vi "AlGaInPAs_v19d.vi"(2 "Debug Mode":bool, 3 "Elapsed Time(s)":dbl, 4 "State":enum16{"Edit", "Start", "Run", "End", "Idle"}(ring), 5 "Argument List In":string[](array[string])) -> (0 "Status Out":string, 1 "Argument List Out":string[](array[string]))   [LabVIEW 2011]
panel:
  out "P bubbler Copy":T1 {"P bubbler main"."Flow" format="%.2f"}
  out "P bubbler":T1 {"P bubbler main"."Flow" format="%.2f"}
  out "As gas Copy":T2 {"As gas main"."Flow" format="%.2f"}
  out "As gas":T2 {"As gas main"."Flow" format="%.2f"}
  out "P gas Copy":T3 {"P gas main"."Flow" format="%.2f"}
  out "P gas":T3 {"P gas main"."Flow" format="%.2f"}
  out "In bubbler Copy":T4 {"In main"."Flow" format="%.2f"}
  in  "In bubbler":T4 {"In main"."Flow" format="%.2f"}
  out "Ga bubbler Copy":T5={"Ga bubbler Active"=FALSE, "Ga main"={"Flow"=0.0, "Ga Run"=FALSE, "Prep Ga"=FALSE, "Dilution"=FALSE, "Ga Calculated"=1, "MFC2 flow"=10.0, "MFC3 flow"=100.0, "MFC1 flow"=0.0}} {"Ga main"."MFC1 flow" format="%.4f"; "Ga main"."MFC3 flow" format="%.1f"; "Ga main"."MFC2 flow" format="%.2f"; "Ga main"."Ga Calculated" items=["Ga flow", "MFC1", "MFC2", "MFC3"]; "Ga main"."Flow" format="%.2f"}
  out "Ga bubbler":T5={"Ga bubbler Active"=FALSE, "Ga main"={"Flow"=0.0, "Ga Run"=FALSE, "Prep Ga"=FALSE, "Dilution"=FALSE, "Ga Calculated"=1, "MFC2 flow"=10.0, "MFC3 flow"=100.0, "MFC1 flow"=0.0}} {"Ga main"."MFC1 flow" format="%.4f"; "Ga main"."MFC3 flow" format="%.1f"; "Ga main"."MFC2 flow" format="%.2f"; "Ga main"."Ga Calculated" items=["Ga flow", "MFC1", "MFC2", "MFC3"]; "Ga main"."Flow" format="%.2f"}
  out "Al bubbler Copy":T6 {"Al main"."Al Flow" format="%.2f"}
  out "Al bubbler":T6 {"Al main"."Al Flow" format="%.2f"}
  out "prep_done":bool
  out "run started":bool
  out "first":bool=TRUE
  out "total time":dbl
  out "is OK?":bool
  in  "prep_time":dbl
  in  "Cancel":bool
  in  "OK":bool
  out "tTotal(s) 2":dbl
  # "Add pre-run time to run time in editor."
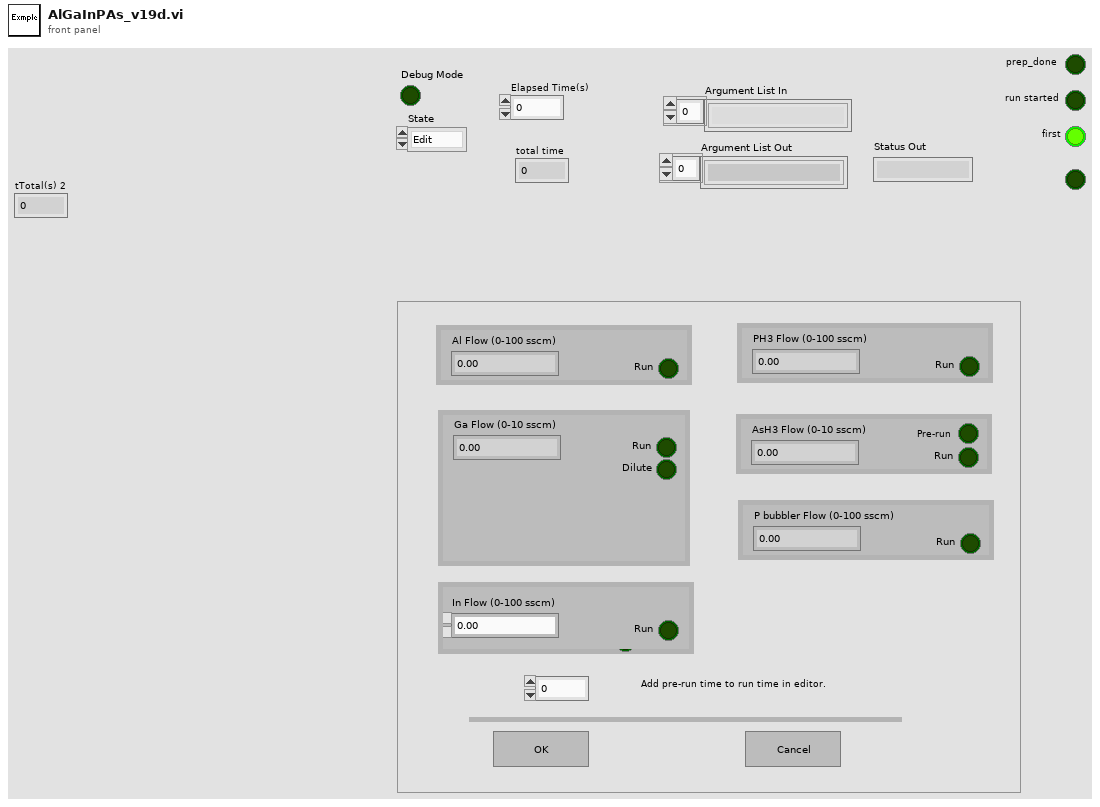
[diagram p1: front panel]
types:
  T1 = cluster{"P bubbler Active":bool, "P bubbler main":cluster{"Flow":dbl, "P bubbler Run":bool, "P bubbler Prep":bool}}
  T2 = cluster{"As gas Active":bool, "As gas main":cluster{"Flow":dbl, "AsH3 Run":bool, "AsH3 Prep":bool}}
  T3 = cluster{"P gas Active":bool, "P gas main":cluster{"Flow":dbl, "PH3 Run":bool, "PH3 Prep":bool}}
  T4 = cluster{"In main":cluster{"Flow":dbl, "In Run":bool, "Prep In":bool}, "In bubbler Active":bool}
  T5 = cluster{"Ga bubbler Active":bool, "Ga main":cluster{"Flow":dbl, "Ga Run":bool, "Prep Ga":bool, "Dilution":bool, "Ga Calculated":u16, "MFC2 flow":dbl, "MFC3 flow":dbl, "MFC1 flow":dbl}}
  T6 = cluster{"Al Active":bool, "Al main":cluster{"Al Flow":dbl, "Al Run":bool, "Prep Al":bool}}
  T7 = enum16{"Discrete", "Continuous", "Instantaneous", "Finite"}
  T8 = enum32{"Invalid", "Default", "Floating", "Floating/Auto-Hide", "Modal"}
  T9 = enum8{"Enabled", "Disabled", "Disabled and Grayed Out"}
  T10 = cluster{"Al Flow":dbl, "Al Run":bool, "Prep Al":bool}
  T11 = cluster{"Flow":dbl, "Ga Run":bool, "Prep Ga":bool, "Dilution":bool, "Ga Calculated":u16, "MFC2 flow":dbl, "MFC3 flow":dbl, "MFC1 flow":dbl}
  T12 = cluster{"Flow":dbl, "In Run":bool, "Prep In":bool}
  T13 = cluster{"Flow":dbl, "PH3 Run":bool, "PH3 Prep":bool}
  T14 = cluster{"Flow":dbl, "AsH3 Run":bool, "AsH3 Prep":bool}
  T15 = cluster{"Flow":dbl, "P bubbler Run":bool, "P bubbler Prep":bool}
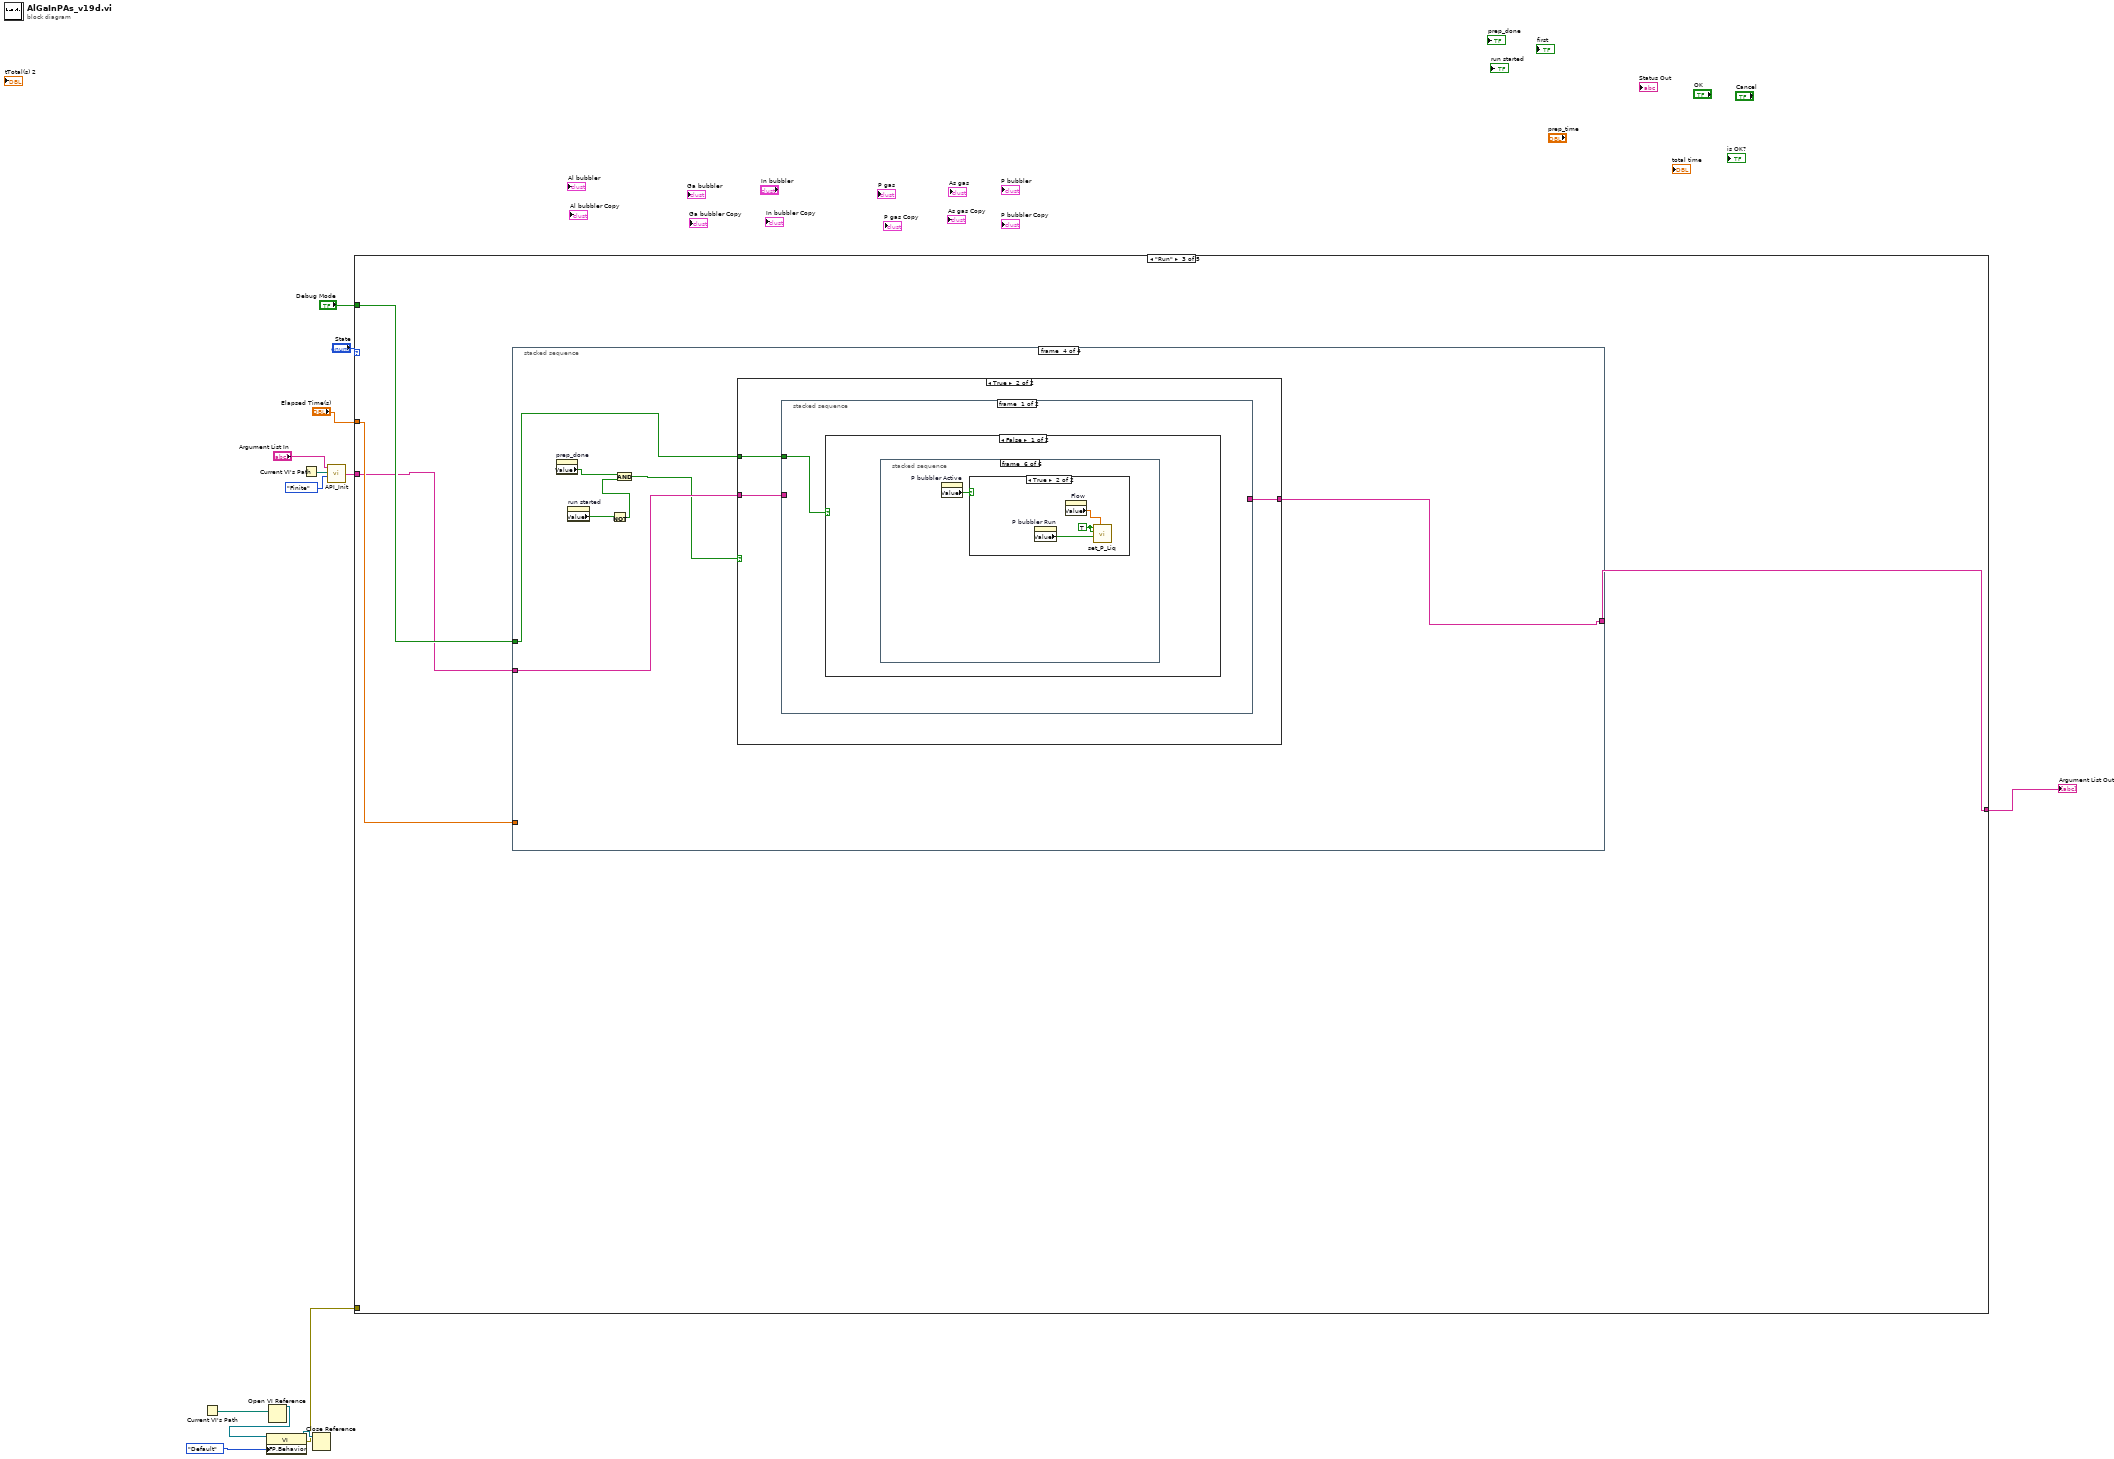
[diagram p0: block diagram]
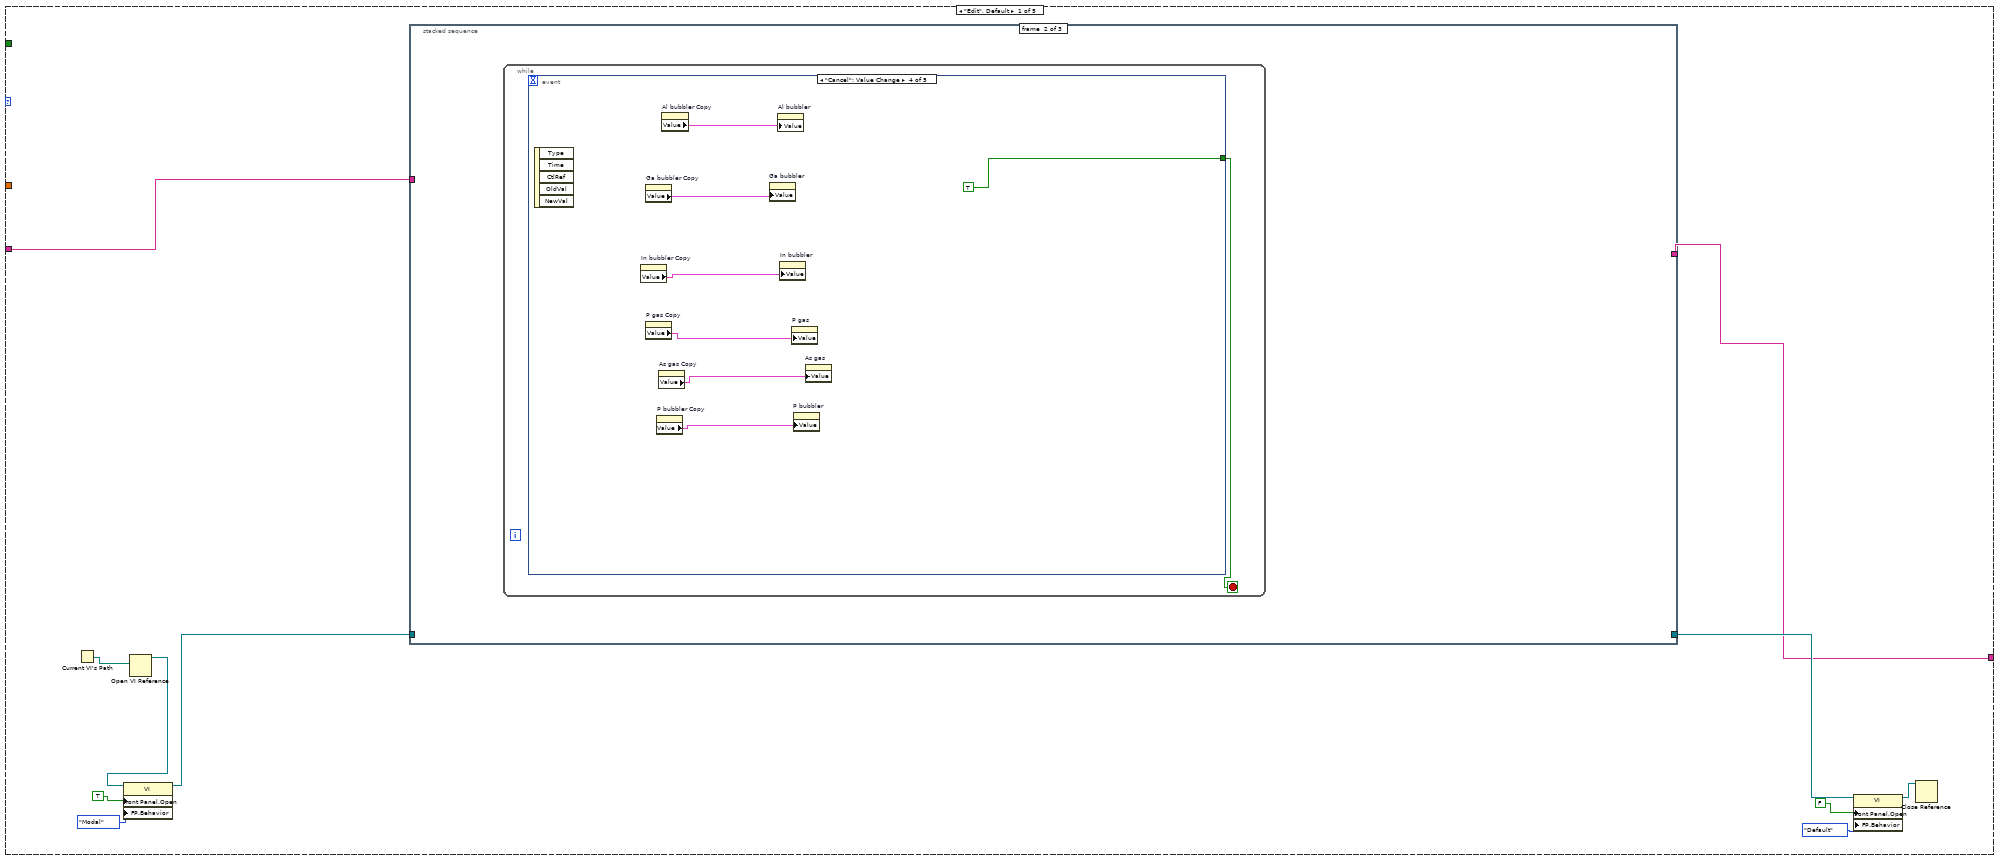
[diagram p2: hidden frame]
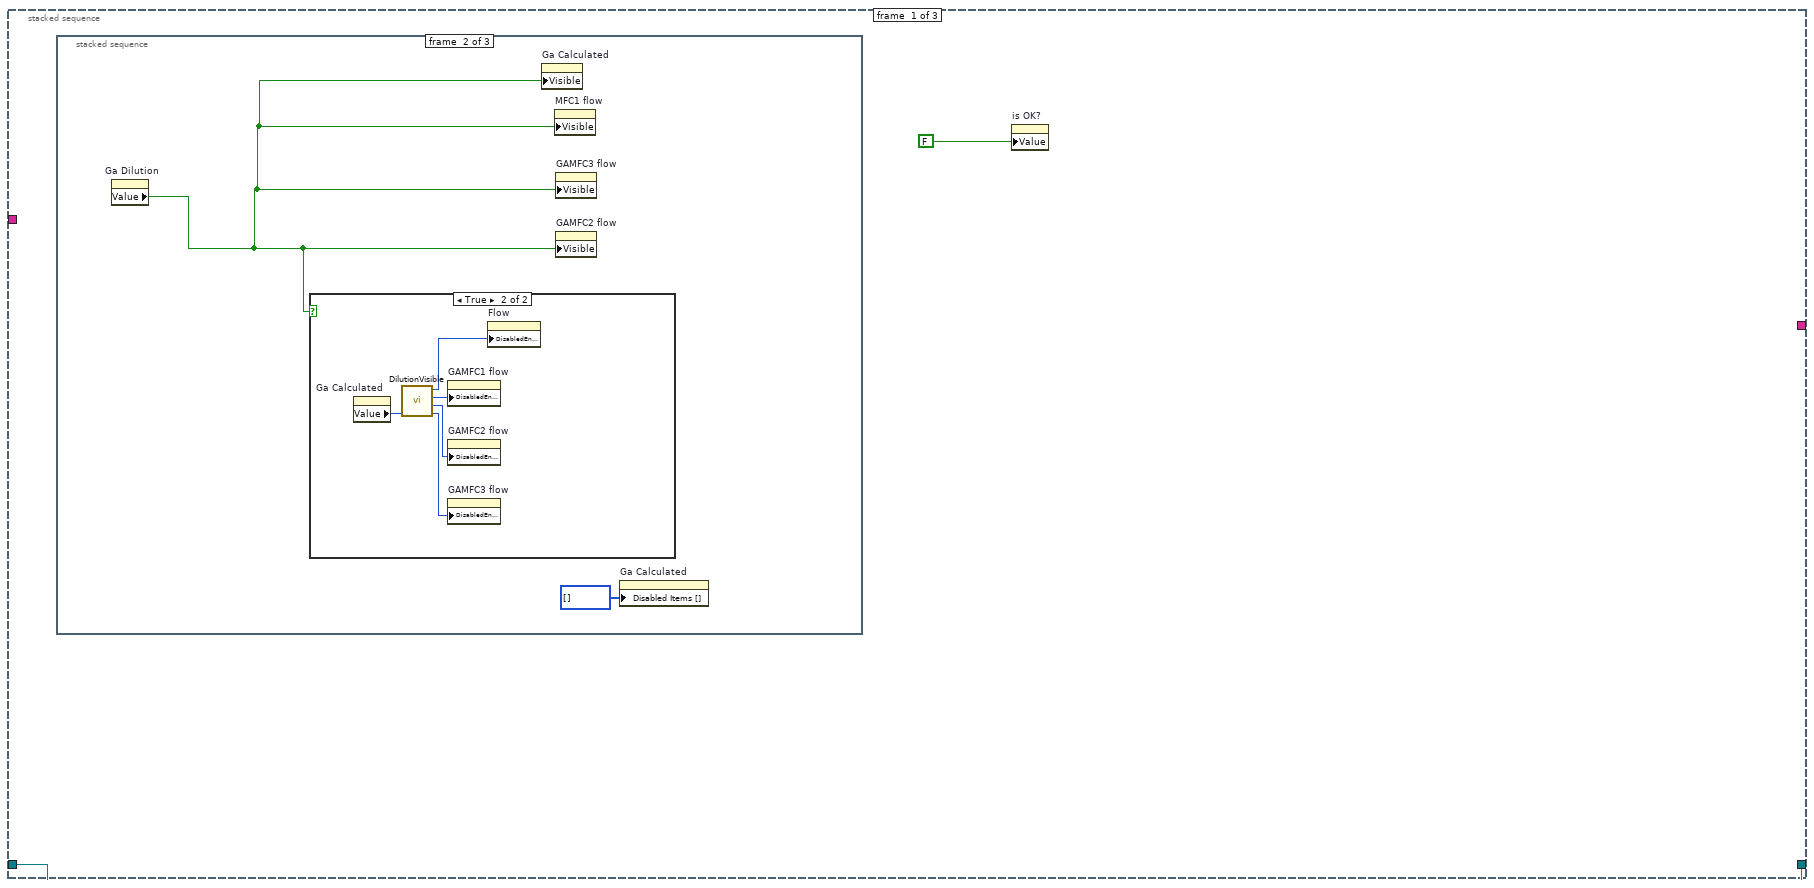
[diagram p3: hidden frame]
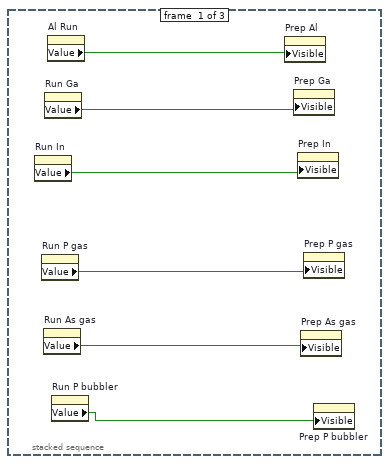
[diagram p4: hidden frame]
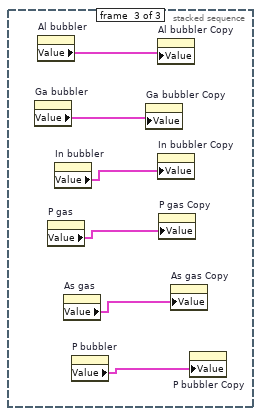
[diagram p6: hidden frame]
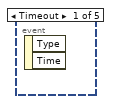
[diagram p7: hidden frame]
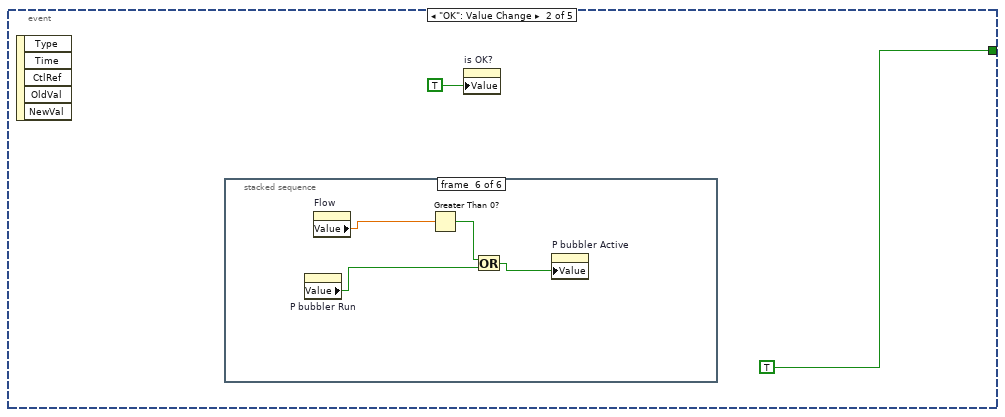
[diagram p8: hidden frame]
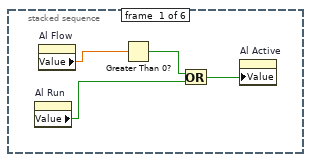
[diagram p9: hidden frame]
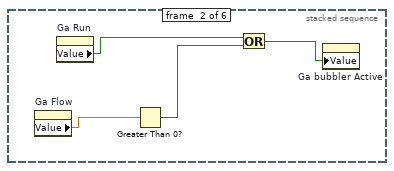
[diagram p10: hidden frame]
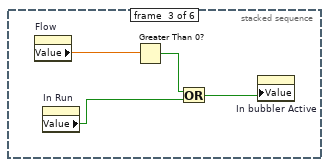
[diagram p11: hidden frame]
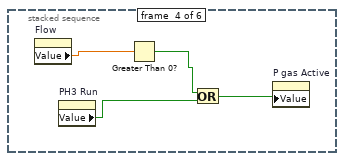
[diagram p12: hidden frame]
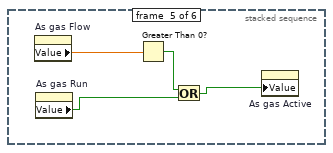
[diagram p13: hidden frame]
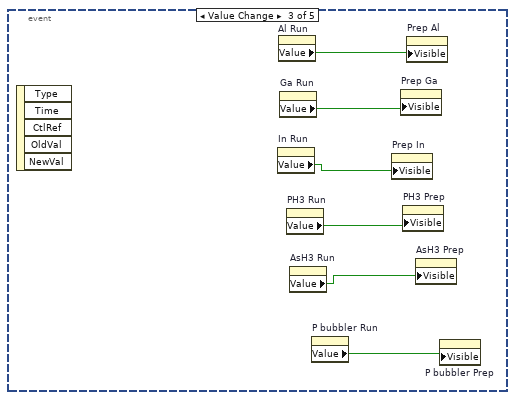
[diagram p14: hidden frame]
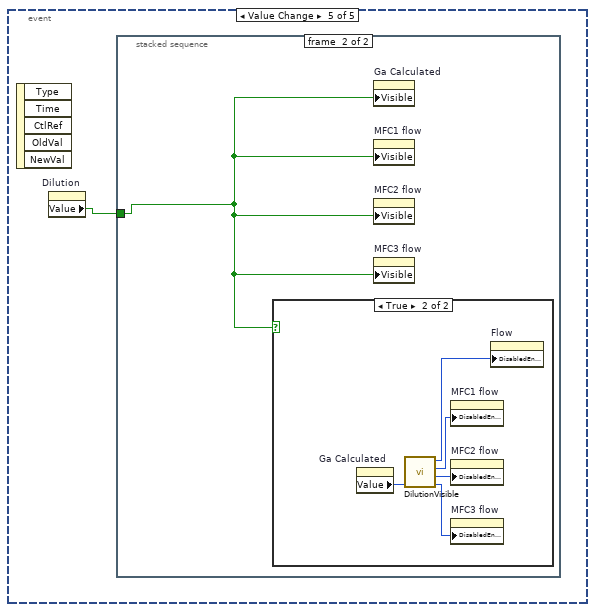
[diagram p15: hidden frame]
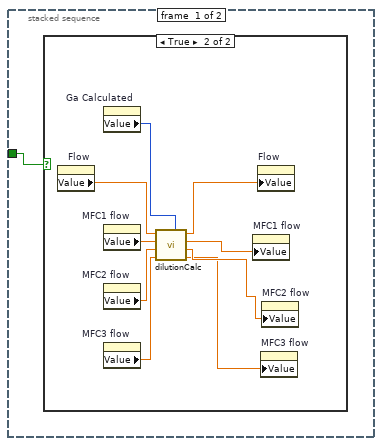
[diagram p16: hidden frame]
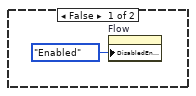
[diagram p18: hidden frame]
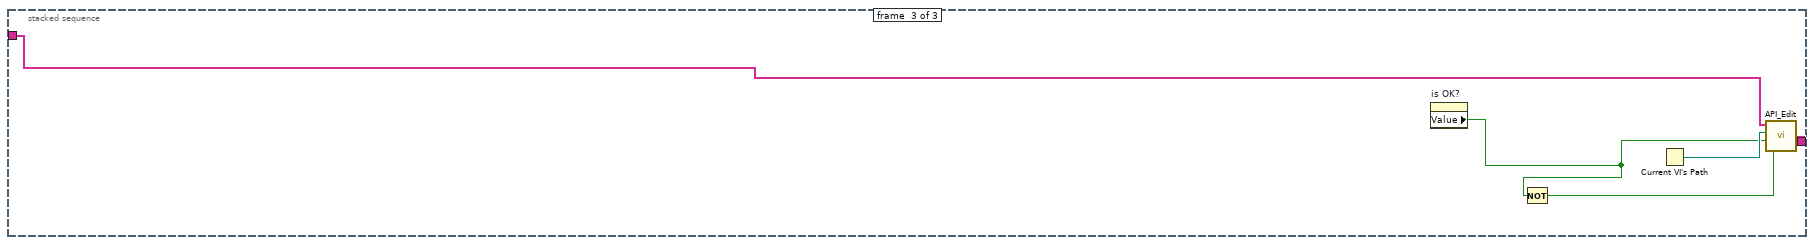
[diagram p19: hidden frame]
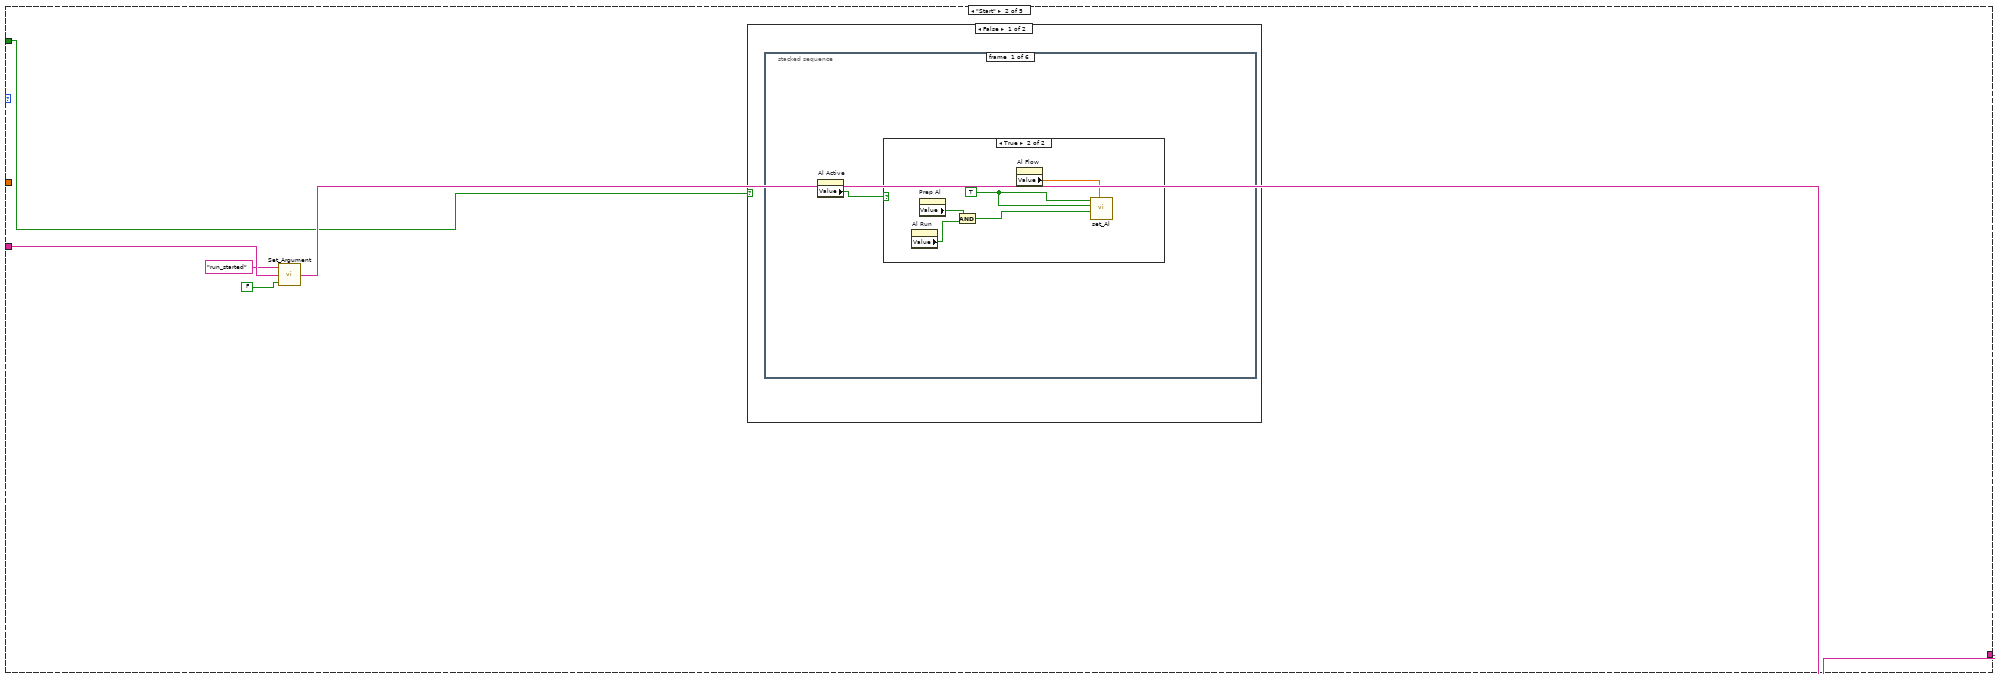
[diagram p20: hidden frame]
diagram:
  n1 = Current VI's Path() -> (path=w9:path)
  n2 = Open VI Reference(vi path=w9) -> (vi reference=w8:refnum<vi>)  [unwired: 1 in, 5 out]
  n3 = property class="VI"(reference=w8, "FP.Behavior"=T8."Default" ("Front Panel Window:Behavior")) -> (reference out=w6:refnum<vi>, error out=w5:errorcluster)  [unwired: 1 in]
  n4 = Current VI's Path() -> (path=w4:path)
  n5 = Close Reference(reference=w6) -> ()  [unwired: 1 in, 1 out]
  n6 = call "API_Init.vi"("API Mode"=T7."Finite", "VI Path"=w4, "Argument List In"="Argument List In") -> ("Argument List Out"=w1:string[])  [unwired: 1 in]
  n7 = case shown="\"Run\"" "State" {
    tunnel: "Debug Mode" -> [_ w109 w167 _ _]
    tunnel: "Elapsed Time(s)" -> [_ _ w168 _ _]
    tunnel: w1 -> [w15 w111 w166 w297 w298]
    tunnel: [w14 w110 w165 w297 w298] -> w10
    tunnel: w5 -> [_ _ _ _ _]
    frame "Edit", Default {
      n8 = Current VI's Path() -> (path=w20:path)
      n9 = Open VI Reference(vi path=w20) -> (vi reference=w19:refnum<vi>)  [unwired: 1 in, 5 out]
      n10 = property class="VI"(reference=w19, "Front Panel.Open"=TRUE ("Front Panel Window:Open"), "FP.Behavior"=T8."Modal" ("Front Panel Window:Behavior")) -> (reference out=w18:refnum<vi>)  [unwired: 1 in, 1 out]
      n11 = stacked-sequence {
        tunnel: w15 -> [_ _ w105]
        tunnel: w18 -> [w26 _ _]
        tunnel: [w26 _ _] -> w22
        tunnel: [_ _ w106] -> w14
        frame #0 {
          n12 = stacked-sequence {
            frame #0 {
              n13 = property on="Run In" class="Bool (strict)"() -> ("Value"=w31:bool)  [unwired: 2 in, 2 out]
              n14 = property on="Run P gas" class="Bool (strict)"() -> ("Value"=w29:bool)  [unwired: 2 in, 2 out]
              n15 = property on="Run As gas" class="Bool (strict)"() -> ("Value"=w28:bool)  [unwired: 2 in, 2 out]
              n16 = property on="Run Ga" class="Bool (strict)"() -> ("Value"=w30:bool)  [unwired: 2 in, 2 out]
              n17 = property on="Al Run" class="Bool (strict)"() -> ("Value"=w32:bool)  [unwired: 2 in, 2 out]
              n18 = property on="Run P bubbler" class="Bool (strict)"() -> ("Value"=w27:bool)  [unwired: 2 in, 2 out]
              n19 = property on="Prep Al" class="Bool (strict)"("Visible"=w32) -> ()  [unwired: 2 in, 2 out]
              n20 = property on="Prep Ga" class="Bool (strict)"("Visible"=w30) -> ()  [unwired: 2 in, 2 out]
              n21 = property on="Prep In" class="Bool (strict)"("Visible"=w31) -> ()  [unwired: 2 in, 2 out]
              n22 = property on="Prep As gas" class="Bool (strict)"("Visible"=w28) -> ()  [unwired: 2 in, 2 out]
              n23 = property on="Prep P gas" class="Bool (strict)"("Visible"=w29) -> ()  [unwired: 2 in, 2 out]
              n24 = property on="Prep P bubbler" class="Bool (strict)"("Visible"=w27) -> ()  [unwired: 2 in, 2 out]
            }
            frame #1 {
              n25 = property on="Ga Dilution" class="Bool (strict)"() -> ("Value"=w34:bool)  [unwired: 2 in, 2 out]
              n26 = case shown="True" w34 {
                frame False {
                }
                frame True {
                  n27 = property on="Ga Calculated" class="Ring (strict)"() -> ("Value"=w35:u16)  [unwired: 2 in, 2 out]
                  n28 = call "DilutionVisible.vi"("calculated"=w35) -> ("MFC3"=w38:u16, "MFC2"=w37:u16, "MFC1"=w36:u16, "flow"=w39:u16)  [unwired: 3 in]
                  n29 = property on="GAMFC1 flow" class="DigNum (strict)"("DisabledEnum"=w36) -> ()  [unwired: 2 in, 2 out]
                  n30 = property on="GAMFC2 flow" class="DigNum (strict)"("DisabledEnum"=w37) -> ()  [unwired: 2 in, 2 out]
                  n31 = property on="GAMFC3 flow" class="DigNum (strict)"("DisabledEnum"=w38) -> ()  [unwired: 2 in, 2 out]
                  n32 = property on="Flow" class="DigNum (strict)"("DisabledEnum"=w39) -> ()  [unwired: 2 in, 2 out]
                }
              }
              n33 = property on="Ga Calculated" class="Ring (strict)"("Visible"=w34) -> ()  [unwired: 2 in, 2 out]
              n34 = property on="MFC1 flow" class="DigNum (strict)"("Visible"=w34) -> ()  [unwired: 2 in, 2 out]
              n35 = property on="GAMFC3 flow" class="DigNum (strict)"("Visible"=w34) -> ()  [unwired: 2 in, 2 out]
              n36 = property on="GAMFC2 flow" class="DigNum (strict)"("Visible"=w34) -> ()  [unwired: 2 in, 2 out]
              n37 = property on="Ga Calculated" class="Ring (strict)"("Disabled Items []"=i32[] []) -> ()  [unwired: 2 in, 2 out]
            }
            frame #2 {
              n38 = property on="Ga bubbler" class="Clust (strict)"() -> ("Value"=w44:T5)  [unwired: 2 in, 2 out]
              n39 = property on="Al bubbler" class="Clust (strict)"() -> ("Value"=w45:T6)  [unwired: 2 in, 2 out]
              n40 = property on="P gas" class="Clust (strict)"() -> ("Value"=w42:T3)  [unwired: 2 in, 2 out]
              n41 = property on="In bubbler" class="Clust (strict)"() -> ("Value"=w43:T4)  [unwired: 2 in, 2 out]
              n42 = property on="As gas" class="Clust (strict)"() -> ("Value"=w41:T2)  [unwired: 2 in, 2 out]
              n43 = property on="P bubbler" class="Clust (strict)"() -> ("Value"=w40:T1)  [unwired: 2 in, 2 out]
              n44 = property on="Ga bubbler Copy" class="Clust (strict)"("Value"=w44) -> ()  [unwired: 2 in, 2 out]
              n45 = property on="Al bubbler Copy" class="Clust (strict)"("Value"=w45) -> ()  [unwired: 2 in, 2 out]
              n46 = property on="In bubbler Copy" class="Clust (strict)"("Value"=w43) -> ()  [unwired: 2 in, 2 out]
              n47 = property on="P gas Copy" class="Clust (strict)"("Value"=w42) -> ()  [unwired: 2 in, 2 out]
              n48 = property on="As gas Copy" class="Clust (strict)"("Value"=w41) -> ()  [unwired: 2 in, 2 out]
              n49 = property on="P bubbler Copy" class="Clust (strict)"("Value"=w40) -> ()  [unwired: 2 in, 2 out]
            }
          }
          n50 = property on="is OK?" class="Bool (strict)"("Value"=FALSE ("is OK?")) -> ()  [unwired: 2 in, 2 out]
        }
        frame #1 {
          n51 = while {
            stop <- w46 stop-if-true
            n52 = event shown="[3] \"Cancel\": Value Change" {
              selector: _ -> [_ _ _ _ _]
              dyn-events: _ -> [_ _ _ _ _]
              timeout: _ -> [_ _ _ _ _]
              tunnel: [_ TRUE _ TRUE _] -> w46
              event Timeout {
                n53 = event-data() -> ()  [unwired: 1 in, 2 out]
              }
              event "OK": Value Change {
                n54 = event-data() -> ()  [unwired: 1 in, 5 out]
                n55 = stacked-sequence {
                  frame #0 {
                    n56 = property on="Al Run" class="Bool (strict)"() -> ("Value"=w50:bool)  [unwired: 2 in, 2 out]
                    n57 = property on="Al Flow" class="DigNum (strict)"() -> ("Value"=w51:dbl)  [unwired: 2 in, 2 out]
                    n58 = Greater Than 0?(x=w51) -> (x > 0?=w52:bool)
                    n59 = Or(x=w52, y=w50) -> (x .or. y?=w49:bool)
                    n60 = property on="Al Active" class="Bool (strict)"("Value"=w49) -> ()  [unwired: 2 in, 2 out]
                  }
                  frame #1 {
                    n61 = property on="Ga Flow" class="DigNum (strict)"() -> ("Value"=w53:dbl)  [unwired: 2 in, 2 out]
                    n62 = property on="Ga Run" class="Bool (strict)"() -> ("Value"=w54:bool)  [unwired: 2 in, 2 out]
                    n63 = Greater Than 0?(x=w53) -> (x > 0?=w56:bool)
                    n64 = Or(x=w54, y=w56) -> (x .or. y?=w55:bool)
                    n65 = property on="Ga bubbler Active" class="Bool (strict)"("Value"=w55) -> ()  [unwired: 2 in, 2 out]
                  }
                  frame #2 {
                    n66 = property on="Flow" class="DigNum (strict)"() -> ("Value"=w59:dbl)  [unwired: 2 in, 2 out]
                    n67 = property on="In Run" class="Bool (strict)"() -> ("Value"=w58:bool)  [unwired: 2 in, 2 out]
                    n68 = Greater Than 0?(x=w59) -> (x > 0?=w60:bool)
                    n69 = Or(x=w60, y=w58) -> (x .or. y?=w57:bool)
                    n70 = property on="In bubbler Active" class="Bool (strict)"("Value"=w57) -> ()  [unwired: 2 in, 2 out]
                  }
                  frame #3 {
                    n71 = property on="Flow" class="DigNum (strict)"() -> ("Value"=w63:dbl)  [unwired: 2 in, 2 out]
                    n72 = property on="PH3 Run" class="Bool (strict)"() -> ("Value"=w62:bool)  [unwired: 2 in, 2 out]
                    n73 = Greater Than 0?(x=w63) -> (x > 0?=w64:bool)
                    n74 = Or(x=w64, y=w62) -> (x .or. y?=w61:bool)
                    n75 = property on="P gas Active" class="Bool (strict)"("Value"=w61) -> ()  [unwired: 2 in, 2 out]
                  }
                  frame #4 {
                    n76 = property on="As gas Flow" class="DigNum (strict)"() -> ("Value"=w67:dbl)  [unwired: 2 in, 2 out]
                    n77 = property on="As gas Run" class="Bool (strict)"() -> ("Value"=w66:bool)  [unwired: 2 in, 2 out]
                    n78 = Greater Than 0?(x=w67) -> (x > 0?=w68:bool)
                    n79 = Or(x=w68, y=w66) -> (x .or. y?=w65:bool)
                    n80 = property on="As gas Active" class="Bool (strict)"("Value"=w65) -> ()  [unwired: 2 in, 2 out]
                  }
                  frame #5 {
                    n81 = property on="P bubbler Run" class="Bool (strict)"() -> ("Value"=w70:bool)  [unwired: 2 in, 2 out]
                    n82 = property on="Flow" class="DigNum (strict)"() -> ("Value"=w71:dbl)  [unwired: 2 in, 2 out]
                    n83 = Greater Than 0?(x=w71) -> (x > 0?=w72:bool)
                    n84 = Or(x=w72, y=w70) -> (x .or. y?=w69:bool)
                    n85 = property on="P bubbler Active" class="Bool (strict)"("Value"=w69) -> ()  [unwired: 2 in, 2 out]
                  }
                }
                n86 = property on="is OK?" class="Bool (strict)"("Value"=TRUE ("is OK?")) -> ()  [unwired: 2 in, 2 out]
              }
              event "Ga bubbler.Ga main.Ga Run", "In bubbler.In main.In Run", "P gas.P gas main.PH3 Run", "As gas.As gas main.AsH3 Run", "Al bubbler.Al main.Al Run", "P bubbler.P bubbler main.P bubbler Run": Value Change {
                n87 = event-data() -> ()  [unwired: 1 in, 5 out]
                n88 = property on="In Run" class="Bool (strict)"() -> ("Value"=w75:bool)  [unwired: 2 in, 2 out]
                n89 = property on="Al Run" class="Bool (strict)"() -> ("Value"=w77:bool)  [unwired: 2 in, 2 out]
                n90 = property on="Ga Run" class="Bool (strict)"() -> ("Value"=w76:bool)  [unwired: 2 in, 2 out]
                n91 = property on="PH3 Run" class="Bool (strict)"() -> ("Value"=w74:bool)  [unwired: 2 in, 2 out]
                n92 = property on="AsH3 Run" class="Bool (strict)"() -> ("Value"=w73:bool)  [unwired: 2 in, 2 out]
                n93 = property on="P bubbler Run" class="Bool (strict)"() -> ("Value"=w78:bool)  [unwired: 2 in, 2 out]
                n94 = property on="Prep In" class="Bool (strict)"("Visible"=w75) -> ()  [unwired: 2 in, 2 out]
                n95 = property on="Prep Ga" class="Bool (strict)"("Visible"=w76) -> ()  [unwired: 2 in, 2 out]
                n96 = property on="PH3 Prep" class="Bool (strict)"("Visible"=w74) -> ()  [unwired: 2 in, 2 out]
                n97 = property on="Prep Al" class="Bool (strict)"("Visible"=w77) -> ()  [unwired: 2 in, 2 out]
                n98 = property on="AsH3 Prep" class="Bool (strict)"("Visible"=w73) -> ()  [unwired: 2 in, 2 out]
                n99 = property on="P bubbler Prep" class="Bool (strict)"("Visible"=w78) -> ()  [unwired: 2 in, 2 out]
              }
              event "Cancel": Value Change {
                n100 = event-data() -> ()  [unwired: 1 in, 5 out]
                n101 = property on="In bubbler Copy" class="Clust (strict)"() -> ("Value"=w83:T4)  [unwired: 2 in, 2 out]
                n102 = property on="Ga bubbler Copy" class="Clust (strict)"() -> ("Value"=w82:T5)  [unwired: 2 in, 2 out]
                n103 = property on="P gas Copy" class="Clust (strict)"() -> ("Value"=w81:T3)  [unwired: 2 in, 2 out]
                n104 = property on="P bubbler Copy" class="Clust (strict)"() -> ("Value"=w79:T1)  [unwired: 2 in, 2 out]
                n105 = property on="As gas Copy" class="Clust (strict)"() -> ("Value"=w80:T2)  [unwired: 2 in, 2 out]
                n106 = property on="Al bubbler Copy" class="Clust (strict)"() -> ("Value"=w84:T6)  [unwired: 2 in, 2 out]
                n107 = property on="Ga bubbler" class="Clust (strict)"("Value"=w82) -> ()  [unwired: 2 in, 2 out]
                n108 = property on="Al bubbler" class="Clust (strict)"("Value"=w84) -> ()  [unwired: 2 in, 2 out]
                n109 = property on="In bubbler" class="Clust (strict)"("Value"=w83) -> ()  [unwired: 2 in, 2 out]
                n110 = property on="P gas" class="Clust (strict)"("Value"=w81) -> ()  [unwired: 2 in, 2 out]
                n111 = property on="P bubbler" class="Clust (strict)"("Value"=w79) -> ()  [unwired: 2 in, 2 out]
                n112 = property on="As gas" class="Clust (strict)"("Value"=w80) -> ()  [unwired: 2 in, 2 out]
              }
              event "Ga bubbler.Ga main.Ga Calculated", "Ga bubbler.Ga main.MFC1 flow", "Ga bubbler.Ga main.MFC2 flow", "Ga bubbler.Ga main.MFC3 flow", "Ga bubbler.Ga main.Flow", "Ga bubbler.Ga main.Dilution": Value Change {
                n113 = event-data() -> ()  [unwired: 1 in, 5 out]
                n114 = property on="Dilution" class="Bool (strict)"() -> ("Value"=w86:bool)  [unwired: 2 in, 2 out]
                n115 = stacked-sequence {
                  tunnel: w86 -> [w87 w97]
                  frame #0 {
                    n116 = case shown="True" w87 {
                      frame False {
                      }
                      frame True {
                        n117 = property on="Flow" class="DigNum (strict)"() -> ("Value"=w95:dbl)  [unwired: 2 in, 2 out]
                        n118 = property on="Ga Calculated" class="Ring (strict)"() -> ("Value"=w96:u16)  [unwired: 2 in, 2 out]
                        n119 = property on="MFC1 flow" class="DigNum (strict)"() -> ("Value"=w94:dbl)  [unwired: 2 in, 2 out]
                        n120 = property on="MFC2 flow" class="DigNum (strict)"() -> ("Value"=w93:dbl)  [unwired: 2 in, 2 out]
                        n121 = property on="MFC3 flow" class="DigNum (strict)"() -> ("Value"=w92:dbl)  [unwired: 2 in, 2 out]
                        n122 = call "dilutionCalc.vi"("Calculated"=w96, "MFC3"=w92, "MFC2"=w93, "MFC1"=w94, "flow"=w95) -> ("MFC3 out"=w88:dbl, "MFC2 out"=w89:dbl, "MFC1 out"=w90:dbl, "flow out"=w91:dbl)  [unwired: 1 in]
                        n123 = property on="MFC1 flow" class="DigNum (strict)"("Value"=w90) -> ()  [unwired: 2 in, 2 out]
                        n124 = property on="Flow" class="DigNum (strict)"("Value"=w91) -> ()  [unwired: 2 in, 2 out]
                        n125 = property on="MFC3 flow" class="DigNum (strict)"("Value"=w88) -> ()  [unwired: 2 in, 2 out]
                        n126 = property on="MFC2 flow" class="DigNum (strict)"("Value"=w89) -> ()  [unwired: 2 in, 2 out]
                      }
                    }
                  }
                  frame #1 {
                    n127 = case shown="True" w97 {
                      frame False {
                        n128 = property on="Flow" class="DigNum (strict)"("DisabledEnum"=T9."Enabled" ("Disabled")) -> ()  [unwired: 2 in, 2 out]
                      }
                      frame True {
                        n129 = property on="Ga Calculated" class="Ring (strict)"() -> ("Value"=w99:u16)  [unwired: 2 in, 2 out]
                        n130 = call "DilutionVisible.vi"("calculated"=w99) -> ("MFC3"=w103:u16, "MFC2"=w102:u16, "MFC1"=w101:u16, "flow"=w100:u16)  [unwired: 3 in]
                        n131 = property on="MFC1 flow" class="DigNum (strict)"("DisabledEnum"=w101) -> ()  [unwired: 2 in, 2 out]
                        n132 = property on="MFC2 flow" class="DigNum (strict)"("DisabledEnum"=w102) -> ()  [unwired: 2 in, 2 out]
                        n133 = property on="MFC3 flow" class="DigNum (strict)"("DisabledEnum"=w103) -> ()  [unwired: 2 in, 2 out]
                        n134 = property on="Flow" class="DigNum (strict)"("DisabledEnum"=w100) -> ()  [unwired: 2 in, 2 out]
                      }
                    }
                    n135 = property on="Ga Calculated" class="Ring (strict)"("Visible"=w97) -> ()  [unwired: 2 in, 2 out]
                    n136 = property on="MFC1 flow" class="DigNum (strict)"("Visible"=w97) -> ()  [unwired: 2 in, 2 out]
                    n137 = property on="MFC2 flow" class="DigNum (strict)"("Visible"=w97) -> ()  [unwired: 2 in, 2 out]
                    n138 = property on="MFC3 flow" class="DigNum (strict)"("Visible"=w97) -> ()  [unwired: 2 in, 2 out]
                  }
                }
              }
            }
          }
        }
        frame #2 {
          n139 = property on="is OK?" class="Bool (strict)"() -> ("Value"=w104:bool)  [unwired: 2 in, 2 out]
          n140 = Not(x=w104) -> (.not. x?=w108:bool)
          n141 = Current VI's Path() -> (path=w107:path)
          n142 = call "API_Edit.vi"("Cancel"=w108, "OK"=w104, "VI Path"=w107, "Argument List In"=w105) -> ("Argument List Out"=w106:string[])
        }
      }
      n143 = property class="VI"(reference=w22, "Front Panel.Open"=FALSE ("Front Panel Window:Open"), "FP.Behavior"=T8."Default" ("Front Panel Window:Behavior")) -> (reference out=w23:refnum<vi>)  [unwired: 1 in, 1 out]
      n144 = Close Reference(reference=w23) -> ()  [unwired: 1 in, 1 out]
    }
    frame "Start" {
      n145 = call "Set_Argument.vi"("Enable"=FALSE, "Argument"="run_started", "Argument List In"=w111) -> ("Argument List Out"=w110:string[])
      n146 = case shown="False" w109 {
        frame False {
          n147 = stacked-sequence {
            frame #0 {
              n148 = property on="Al Active" class="Bool (strict)"() -> ("Value"=w114:bool)  [unwired: 2 in, 2 out]
              n149 = case shown="True" w114 {
                frame False {
                  w115 = FALSE ("Al Active")
                  n150 = call "set_Al.vi"("ALMFC1"=0.0 ("Aluminum Flow"), "Remote"=w115, "Run"=w115, "Bubbler In"=w115, "Active"=w115) -> ()  [unwired: 5 out]
                }
                frame True {
                  w121 = TRUE ("Al Active")
                  n151 = property on="Al Run" class="Bool (strict)"() -> ("Value"=w117:bool)  [unwired: 2 in, 2 out]
                  n152 = property on="Prep Al" class="Bool (strict)"() -> ("Value"=w118:bool)  [unwired: 2 in, 2 out]
                  n153 = And(x=w118, y=w117) -> (x .and. y?=w120:bool)
                  n154 = property on="Al Flow" class="DigNum (strict)"() -> ("Value"=w119:dbl)  [unwired: 2 in, 2 out]
                  n155 = call "set_Al.vi"("ALMFC1"=w119, "Run"=w120, "Bubbler In"=w121, "Active"=w121) -> ()  [unwired: 1 in, 5 out]
                }
              }
            }
            frame #1 {
              n156 = property on="Ga bubbler Active" class="Bool (strict)"() -> ("Value"=w122:bool)  [unwired: 2 in, 2 out]
              n157 = case shown="True" w122 {
                frame False {
                  w124 = FALSE ("Ga Active")
                  w123 = 0.0 ("Ga Flow 1")
                  n158 = call "set_Ga.vi"("Active"=w124, "GAMFC3"=w123, "GAMFC2"=w123, "GAMFC1"=w123, "Bubbler In"=w124, "H2 Dilute"=w124, "Run"=w124, "Remote"=w124) -> ()  [unwired: 8 out]
                }
                frame True {
                  w131 = TRUE ("Ga Active")
                  n159 = property on="Prep Ga" class="Bool (strict)"() -> ("Value"=w128:bool)  [unwired: 2 in, 2 out]
                  n160 = property on="Dilution" class="Bool (strict)"() -> ("Value"=w130:bool)  [unwired: 2 in, 2 out]
                  n161 = property on="MFC1 flow" class="DigNum (strict)"() -> ("Value"=w127:dbl)  [unwired: 2 in, 2 out]
                  n162 = property on="Ga Run" class="Bool (strict)"() -> ("Value"=w129:bool)  [unwired: 2 in, 2 out]
                  n163 = And(x=w128, y=w129) -> (x .and. y?=w132:bool)
                  n164 = property on="MFC2 flow" class="DigNum (strict)"() -> ("Value"=w126:dbl)  [unwired: 2 in, 2 out]
                  n165 = property on="MFC3 flow" class="DigNum (strict)"() -> ("Value"=w125:dbl)  [unwired: 2 in, 2 out]
                  n166 = call "set_Ga.vi"("Active"=w131, "GAMFC3"=w125, "GAMFC2"=w126, "GAMFC1"=w127, "Bubbler In"=w131, "H2 Dilute"=w130, "Run"=w132, "Remote"=w131) -> ()  [unwired: 8 in]
                }
              }
            }
            frame #2 {
              n167 = property on="In bubbler Active" class="Bool (strict)"() -> ("Value"=w133:bool)  [unwired: 2 in, 2 out]
              n168 = case shown="False" w133 {
                frame False {
                  w135 = FALSE ("In Remote")
                  n169 = call "set_In.vi"("INMFC1"=0.0 ("Indium Flow"), "Remote"=w135, "Run"=w135, "Bubbler In"=w135, "Active"=w135) -> ()  [unwired: 5 out]
                }
                frame True {
                  w140 = TRUE ("In Run")
                  n170 = property on="In Run" class="Bool (strict)"() -> ("Value"=w137:bool)  [unwired: 2 in, 2 out]
                  n171 = property on="Prep In" class="Bool (strict)"() -> ("Value"=w138:bool)  [unwired: 2 in, 2 out]
                  n172 = And(x=w137, y=w138) -> (x .and. y?=w139:bool)
                  n173 = property on="Flow" class="DigNum (strict)"() -> ("Value"=w136:dbl)  [unwired: 2 in, 2 out]
                  n174 = call "set_In.vi"("INMFC1"=w136, "Run"=w139, "Bubbler In"=w140, "Active"=w140) -> ()  [unwired: 1 in, 5 out]
                }
              }
            }
            frame #3 {
              n175 = property on="P gas Active" class="Bool (strict)"() -> ("Value"=w141:bool)  [unwired: 2 in, 2 out]
              n176 = case shown="False" w141 {
                frame False {
                  w142 = FALSE ("P_Gas Active")
                  n177 = call "set_P_gas.vi"("Run"=w142, "Gas In"=w142, "Active"=w142, "P_Gas Remote"=w142, "H2 Flush"=w142, "P_Gas Flow"=0.0) -> ()
                }
                frame True {
                  w148 = TRUE ("P_Gas Active")
                  n178 = property on="Flow" class="DigNum (strict)"() -> ("Value"=w146:dbl)  [unwired: 2 in, 2 out]
                  n179 = property on="PH3 Prep" class="Bool (strict)"() -> ("Value"=w145:bool)  [unwired: 2 in, 2 out]
                  n180 = property on="PH3 Run" class="Bool (strict)"() -> ("Value"=w144:bool)  [unwired: 2 in, 2 out]
                  n181 = And(x=w145, y=w144) -> (x .and. y?=w147:bool)
                  n182 = call "set_P_gas.vi"("Active"=w148, "P_Gas Remote"=w147, "H2 Flush"=w148, "P_Gas Flow"=w146) -> ()  [unwired: 2 in]
                }
              }
            }
            frame #4 {
              n183 = property on="As gas Active" class="Bool (strict)"() -> ("Value"=w149:bool)  [unwired: 2 in, 2 out]
              n184 = case shown="False" w149 {
                frame False {
                  w150 = FALSE ("As_Gas Active")
                  n185 = call "set_As_gas.vi"("Active"=w150, "As_Gas Flow"=0.0, "Gas In"=w150, "H2 Flush"=w150, "Run"=w150, "Remote"=w150) -> ()  [unwired: 10 in]
                }
                frame True {
                  w156 = TRUE ("As_Gas Active")
                  n186 = property on="AsH3 Run" class="Bool (strict)"() -> ("Value"=w152:bool)  [unwired: 2 in, 2 out]
                  n187 = property on="AsH3 Prep" class="Bool (strict)"() -> ("Value"=w153:bool)  [unwired: 2 in, 2 out]
                  n188 = And(x=w153, y=w152) -> (x .and. y?=w155:bool)
                  n189 = property on="Flow" class="DigNum (strict)"() -> ("Value"=w154:dbl)  [unwired: 2 in, 2 out]
                  n190 = call "set_As_gas.vi"("Active"=w156, "As_Gas Flow"=w154, "Gas In"=w156, "Run"=w155) -> ()  [unwired: 12 in]
                }
              }
            }
            frame #5 {
              n191 = property on="P bubbler Active" class="Bool (strict)"() -> ("Value"=w157:bool)  [unwired: 2 in, 2 out]
              n192 = case shown="False" w157 {
                frame False {
                  w158 = FALSE ("As_Gas Active")
                  n193 = call "set_P_Liq.vi"("flow 1"=0.0 ("As_Gas Flow"), "Remote"=w158, "Run"=w158, "Bubbler In"=w158, "Active"=w158) -> ()  [unwired: 5 in]
                }
                frame True {
                  w164 = TRUE ("As_Gas Active")
                  n194 = property on="P bubbler Run" class="Bool (strict)"() -> ("Value"=w160:bool)  [unwired: 2 in, 2 out]
                  n195 = property on="P bubbler Prep" class="Bool (strict)"() -> ("Value"=w161:bool)  [unwired: 2 in, 2 out]
                  n196 = And(x=w161, y=w160) -> (x .and. y?=w163:bool)
                  n197 = property on="Flow" class="DigNum (strict)"() -> ("Value"=w162:dbl)  [unwired: 2 in, 2 out]
                  n198 = call "set_P_Liq.vi"("flow 1"=w162, "Run"=w163, "Bubbler In"=w164, "Active"=w164) -> ()  [unwired: 6 in]
                }
              }
            }
          }
        }
        frame True {
        }
      }
    }
    frame "Run" {
      n199 = stacked-sequence {
        tunnel: w168 -> [_ w173 _ _]
        tunnel: w166 -> [w170 _ _ w244]
        tunnel: w167 -> [_ _ _ w242]
        tunnel: [_ _ _ w243] -> w165
        frame #0 {
          n200 = call "Get_Argument.vi"("Argument"="run_started", "Argument List"=w170) -> ("Enabled"=w169:bool)
          n201 = local write "run started"(w169) -> ()
        }
        frame #1 {
          n202 = property on="prep_time" class="DigNum (strict)"() -> ("Value"=w174:dbl)  [unwired: 2 in, 2 out]
          n203 = Greater Or Equal?(x=w173, y=w174) -> (x >= y?=w172:bool)
          n204 = local write "prep_done"(w172) -> ()
        }
        frame #2 {
          n205 = local read "run started"() -> (w176:bool)
          n206 = Not(x=w176) -> (.not. x?=w175:bool)
          n207 = stacked-sequence {
            tunnel: w175 -> [w178 w185 w195 w205 w215 w225 w235]
            frame #0 {
              n208 = case shown="False" w178 {
                tunnel: ["run: " "pre-run: "] -> w177
                frame False {
                }
                frame True {
                }
              }
              n209 = property on="Status Out" class="Str"("Value"=w177) -> ()  [unwired: 2 in, 2 out]
            }
            frame #1 {
              n210 = property on="Al main" class="Clust (strict)"() -> ("Value"=w183:T10)  [unwired: 2 in, 2 out]
              n211 = property on="Al Active" class="Bool (strict)"() -> ("Value"=w184:bool)  [unwired: 2 in, 2 out]
              n212 = property on="Status Out" class="Str"() -> ("Value"=w190:string)  [unwired: 2 in, 2 out]
              n213 = Unbundle By Name(w183) -> ("Al Run"=w182:bool, "Prep Al"=w181:bool)
              n214 = call "flow_strings.vi"("string in"=w190, "is first in?"=TRUE, "use source?"=w184, "name"="Al", "run source?"=w182, "prep source?"=w181, "is prep?"=w185) -> ("string out"=w189:string, "is first out?"=w188:bool)
              n215 = property on="Status Out" class="Str"("Value"=w189) -> ()  [unwired: 2 in, 2 out]
              n216 = property on="first" class="Bool (strict)"("Value"=w188) -> ()  [unwired: 2 in, 2 out]
            }
            frame #2 {
              n217 = property on="Ga main" class="Clust (strict)"() -> ("Value"=w193:T11)  [unwired: 2 in, 2 out]
              n218 = property on="Ga bubbler Active" class="Bool (strict)"() -> ("Value"=w194:bool)  [unwired: 2 in, 2 out]
              n219 = property on="first" class="Bool (strict)"() -> ("Value"=w197:bool)  [unwired: 2 in, 2 out]
              n220 = property on="Status Out" class="Str"() -> ("Value"=w199:string)  [unwired: 2 in, 2 out]
              n221 = Unbundle By Name(w193) -> ("Ga Run"=w192:bool, "Prep Ga"=w191:bool)
              n222 = call "flow_strings.vi"("string in"=w199, "is first in?"=w197, "use source?"=w194, "name"="Ga", "run source?"=w192, "prep source?"=w191, "is prep?"=w195) -> ("string out"=w200:string, "is first out?"=w196:bool)
              n223 = property on="Status Out" class="Str"("Value"=w200) -> ()  [unwired: 2 in, 2 out]
              n224 = property on="first" class="Bool (strict)"("Value"=w196) -> ()  [unwired: 2 in, 2 out]
            }
            frame #3 {
              n225 = property on="In bubbler Active" class="Bool (strict)"() -> ("Value"=w204:bool)  [unwired: 2 in, 2 out]
              n226 = property on="In main" class="Clust (strict)"() -> ("Value"=w203:T12)  [unwired: 2 in, 2 out]
              n227 = property on="first" class="Bool (strict)"() -> ("Value"=w208:bool)  [unwired: 2 in, 2 out]
              n228 = property on="Status Out" class="Str"() -> ("Value"=w210:string)  [unwired: 2 in, 2 out]
              n229 = Unbundle By Name(w203) -> ("In Run"=w202:bool, "Prep In"=w201:bool)
              n230 = call "flow_strings.vi"("string in"=w210, "is first in?"=w208, "use source?"=w204, "name"="In", "run source?"=w202, "prep source?"=w201, "is prep?"=w205) -> ("string out"=w207:string, "is first out?"=w206:bool)
              n231 = property on="Status Out" class="Str"("Value"=w207) -> ()  [unwired: 2 in, 2 out]
              n232 = property on="first" class="Bool (strict)"("Value"=w206) -> ()  [unwired: 2 in, 2 out]
            }
            frame #4 {
              n233 = property on="P gas Active" class="Bool (strict)"() -> ("Value"=w214:bool)  [unwired: 2 in, 2 out]
              n234 = property on="P gas main" class="Clust (strict)"() -> ("Value"=w213:T13)  [unwired: 2 in, 2 out]
              n235 = property on="first" class="Bool (strict)"() -> ("Value"=w217:bool)  [unwired: 2 in, 2 out]
              n236 = property on="Status Out" class="Str"() -> ("Value"=w219:string)  [unwired: 2 in, 2 out]
              n237 = Unbundle By Name(w213) -> ("PH3 Run"=w212:bool, "PH3 Prep"=w211:bool)
              n238 = call "flow_strings.vi"("string in"=w219, "is first in?"=w217, "use source?"=w214, "name"="PH3", "run source?"=w212, "prep source?"=w211, "is prep?"=w215) -> ("string out"=w218:string, "is first out?"=w216:bool)
              n239 = property on="Status Out" class="Str"("Value"=w218) -> ()  [unwired: 2 in, 2 out]
              n240 = property on="first" class="Bool (strict)"("Value"=w216) -> ()  [unwired: 2 in, 2 out]
            }
            frame #5 {
              n241 = property on="As gas Active" class="Bool (strict)"() -> ("Value"=w224:bool)  [unwired: 2 in, 2 out]
              n242 = property on="As gas main" class="Clust (strict)"() -> ("Value"=w223:T14)  [unwired: 2 in, 2 out]
              n243 = property on="first" class="Bool (strict)"() -> ("Value"=w227:bool)  [unwired: 2 in, 2 out]
              n244 = property on="Status Out" class="Str"() -> ("Value"=w229:string)  [unwired: 2 in, 2 out]
              n245 = Unbundle By Name(w223) -> ("AsH3 Run"=w222:bool, "AsH3 Prep"=w221:bool)
              n246 = call "flow_strings.vi"("string in"=w229, "is first in?"=w227, "use source?"=w224, "name"="AsH3", "run source?"=w222, "prep source?"=w221, "is prep?"=w225) -> ("string out"=w226:string, "is first out?"=w228:bool)
              n247 = property on="Status Out" class="Str"("Value"=w226) -> ()  [unwired: 2 in, 2 out]
              n248 = property on="first" class="Bool (strict)"("Value"=w228) -> ()  [unwired: 2 in, 2 out]
            }
            frame #6 {
              n249 = property on="P bubbler main" class="Clust (strict)"() -> ("Value"=w233:T15)  [unwired: 2 in, 2 out]
              n250 = property on="P bubbler Active" class="Bool (strict)"() -> ("Value"=w234:bool)  [unwired: 2 in, 2 out]
              n251 = Unbundle By Name(w233) -> ("P bubbler Run"=w232:bool, "P bubbler Prep"=w231:bool)
              n252 = property on="first" class="Bool (strict)"() -> ("Value"=w238:bool)  [unwired: 2 in, 2 out]
              n253 = property on="Status Out" class="Str"() -> ("Value"=w240:string)  [unwired: 2 in, 2 out]
              n254 = call "flow_strings.vi"("string in"=w240, "is first in?"=w238, "use source?"=w234, "name"="P liq", "run source?"=w232, "prep source?"=w231, "is prep?"=w235) -> ("string out"=w237:string, "is first out?"=w236:bool)
              n255 = property on="Status Out" class="Str"("Value"=w237) -> ()  [unwired: 2 in, 2 out]
              n256 = property on="first" class="Bool (strict)"("Value"=w236) -> ()  [unwired: 2 in, 2 out]
            }
          }
        }
        frame #3 {
          n257 = property on="prep_done" class="Bool (strict)"() -> ("Value"=w247:bool)  [unwired: 2 in, 2 out]
          n258 = property on="run started" class="Bool (strict)"() -> ("Value"=w246:bool)  [unwired: 2 in, 2 out]
          n259 = Not(x=w246) -> (.not. x?=w245:bool)
          n260 = And(x=w247, y=w245) -> (x .and. y?=w241:bool)
          n261 = case shown="True" w241 {
            tunnel: w244 -> [w248 w251]
            tunnel: [w248 w250] -> w243
            tunnel: w242 -> [_ w249]
            frame False {
            }
            frame True {
              n262 = stacked-sequence {
                tunnel: w249 -> [w252 _]
                tunnel: w251 -> [_ w294]
                tunnel: [_ w293] -> w250
                frame #0 {
                  n263 = case shown="False" w252 {
                    frame False {
                      n264 = stacked-sequence {
                        frame #0 {
                          n265 = property on="Al Active" class="Bool (strict)"() -> ("Value"=w253:bool)  [unwired: 2 in, 2 out]
                          n266 = case shown="True" w253 {
                            frame False {
                              w254 = FALSE ("Al Active")
                              n267 = call "set_Al.vi"("ALMFC1"=0.0 ("Aluminum Flow"), "Remote"=w254, "Run"=w254, "Bubbler In"=w254, "Active"=w254) -> ()  [unwired: 5 out]
                            }
                            frame True {
                              w258 = TRUE ("Al Active")
                              n268 = property on="Al Flow" class="DigNum (strict)"() -> ("Value"=w257:dbl)  [unwired: 2 in, 2 out]
                              n269 = property on="Al Run" class="Bool (strict)"() -> ("Value"=w256:bool)  [unwired: 2 in, 2 out]
                              n270 = call "set_Al.vi"("ALMFC1"=w257, "Run"=w256, "Bubbler In"=w258, "Active"=w258) -> ()  [unwired: 1 in, 5 out]
                            }
                          }
                        }
                        frame #1 {
                          n271 = property on="Ga bubbler Active" class="Bool (strict)"() -> ("Value"=w259:bool)  [unwired: 2 in, 2 out]
                          n272 = case shown="True" w259 {
                            frame False {
                              w261 = FALSE ("Ga Active")
                              w260 = 0.0 ("Ga Flow 1")
                              n273 = call "set_Ga.vi"("Active"=w261, "GAMFC3"=w260, "GAMFC2"=w260, "GAMFC1"=w260, "Bubbler In"=w261, "H2 Dilute"=w261, "Run"=w261, "Remote"=w261) -> ()  [unwired: 8 out]
                            }
                            frame True {
                              w267 = TRUE ("Ga Active")
                              n274 = property on="MFC1 flow" class="DigNum (strict)"() -> ("Value"=w264:dbl)  [unwired: 2 in, 2 out]
                              n275 = property on="MFC2 flow" class="DigNum (strict)"() -> ("Value"=w263:dbl)  [unwired: 2 in, 2 out]
                              n276 = property on="MFC3 flow" class="DigNum (strict)"() -> ("Value"=w262:dbl)  [unwired: 2 in, 2 out]
                              n277 = property on="Dilution" class="Bool (strict)"() -> ("Value"=w265:bool)  [unwired: 2 in, 2 out]
                              n278 = property on="Ga Run" class="Bool (strict)"() -> ("Value"=w266:bool)  [unwired: 2 in, 2 out]
                              n279 = call "set_Ga.vi"("Active"=w267, "GAMFC3"=w262, "GAMFC2"=w263, "GAMFC1"=w264, "Bubbler In"=w267, "H2 Dilute"=w265, "Run"=w266, "Remote"=w267) -> ()  [unwired: 8 in]
                            }
                          }
                        }
                        frame #2 {
                          n280 = property on="In bubbler Active" class="Bool (strict)"() -> ("Value"=w268:bool)  [unwired: 2 in, 2 out]
                          n281 = case shown="True" w268 {
                            frame False {
                              w270 = FALSE ("In Remote")
                              n282 = call "set_In.vi"("INMFC1"=0.0 ("Indium Flow"), "Remote"=w270, "Run"=w270, "Bubbler In"=w270, "Active"=w270) -> ()  [unwired: 5 out]
                            }
                            frame True {
                              w273 = TRUE ("In Run")
                              n283 = property on="In Run" class="Bool (strict)"() -> ("Value"=w271:bool)  [unwired: 2 in, 2 out]
                              n284 = property on="In Flow" class="DigNum (strict)"() -> ("Value"=w272:dbl)  [unwired: 2 in, 2 out]
                              n285 = call "set_In.vi"("INMFC1"=w272, "Run"=w271, "Bubbler In"=w273, "Active"=w273) -> ()  [unwired: 1 in, 5 out]
                            }
                          }
                        }
                        frame #3 {
                          n286 = property on="P gas Active" class="Bool (strict)"() -> ("Value"=w274:bool)  [unwired: 2 in, 2 out]
                          n287 = case shown="False" w274 {
                            frame False {
                              w275 = FALSE ("P_Gas Active")
                              n288 = call "set_P_gas.vi"("Run"=w275, "Gas In"=w275, "Active"=w275, "P_Gas Remote"=w275, "H2 Flush"=w275, "P_Gas Flow"=0.0) -> ()
                            }
                            frame True {
                              n289 = property on="Flow" class="DigNum (strict)"() -> ("Value"=w279:dbl)  [unwired: 2 in, 2 out]
                              n290 = property on="PH3 Run" class="Bool (strict)"() -> ("Value"=w278:bool)  [unwired: 2 in, 2 out]
                              n291 = call "set_P_gas.vi"("Run"=w278, "Gas In"=TRUE, "Active"=TRUE ("P_Gas Active"), "P_Gas Flow"=w279) -> ()  [unwired: 2 in]
                            }
                          }
                        }
                        frame #4 {
                          n292 = property on="As gas Active" class="Bool (strict)"() -> ("Value"=w281:bool)  [unwired: 2 in, 2 out]
                          n293 = case shown="True" w281 {
                            frame False {
                              w282 = FALSE ("As_Gas Active")
                              n294 = call "set_As_gas.vi"("Active"=w282, "As_Gas Flow"=0.0, "Gas In"=w282, "H2 Flush"=w282, "Run"=w282, "Remote"=w282) -> ()  [unwired: 10 in]
                            }
                            frame True {
                              w286 = TRUE ("As_Gas Active")
                              n295 = property on="Flow" class="DigNum (strict)"() -> ("Value"=w284:dbl)  [unwired: 2 in, 2 out]
                              n296 = property on="AsH3 Run" class="Bool (strict)"() -> ("Value"=w285:bool)  [unwired: 2 in, 2 out]
                              n297 = call "set_As_gas.vi"("Active"=w286, "As_Gas Flow"=w284, "Gas In"=w286, "Run"=w285) -> ()  [unwired: 12 in]
                            }
                          }
                        }
                        frame #5 {
                          n298 = property on="P bubbler Active" class="Bool (strict)"() -> ("Value"=w287:bool)  [unwired: 2 in, 2 out]
                          n299 = case shown="True" w287 {
                            frame False {
                              w289 = FALSE ("In Remote")
                              n300 = call "set_P_Liq.vi"("flow 1"=0.0 ("Indium Flow"), "Remote"=w289, "Run"=w289, "Bubbler In"=w289, "Active"=w289) -> ()  [unwired: 5 in]
                            }
                            frame True {
                              w292 = TRUE ("In Run")
                              n301 = property on="P bubbler Run" class="Bool (strict)"() -> ("Value"=w290:bool)  [unwired: 2 in, 2 out]
                              n302 = property on="Flow" class="DigNum (strict)"() -> ("Value"=w291:dbl)  [unwired: 2 in, 2 out]
                              n303 = call "set_P_Liq.vi"("flow 1"=w291, "Run"=w290, "Bubbler In"=w292, "Active"=w292) -> ()  [unwired: 6 in]
                            }
                          }
                        }
                      }
                    }
                    frame True {
                    }
                  }
                }
                frame #1 {
                  n304 = call "Set_Argument.vi"("Enable"=TRUE, "Argument"="run_started", "Argument List In"=w294) -> ("Argument List Out"=w293:string[])
                }
              }
            }
          }
        }
      }
    }
    frame "End" {
    }
    frame "Idle" {
    }
  }
  "Argument List Out" <- w10
